vi "Rotate pi.vi"(11 "Degrees":dbl=180.0 format="%#_13g") -> ()   [LabVIEW 2015]
doc: "Assumes that + rotation is clockwise and - is counterclockwise"
uses:
  Sprocket/src/Action/Action Name.ctl
  Sprocket/src/Refname/Refname to String.vi
  Sprocket/src/Refname/Refname to String (Queue).vi
  Sprocket/src/Stream/Obtain Stream.vi
  Sprocket/src/Stream/Push Stream.vi
  Sprocket/src/Stream/Release Stream.vi
  Sprocket/lib/Sprocket.lvlib
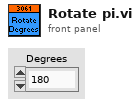
[diagram p1: front panel]
types:
  T1 = typedef "Sprocket.lvlib/Action Name.ctl" = enum16{"No Action", "Drive Train Both", "Drive Train Rotate", "Drive Train Throttle", "Collector Motor Roll", "Collector Motor Eject", "Collector Motor Collect", "Collector Motor Stop", "Collector Extend", "Collector Retract", "Shifter High", "Shifter Low", "Collector Motor Stall", "Wedge Roll"}
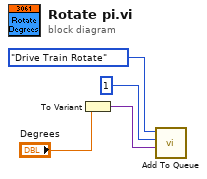
[diagram p0: block diagram]
diagram:
  n1 = To Variant(anything="Degrees") -> (Variant=w2:variant)
  n2 = call "Add To Queue.vi"("Data"=w2, "Priority"=1, "Action"=Action_Name."Drive Train Rotate") -> ()  [unwired: 8 in, 1 out]
